vi "Escribir TDMS Parametro Meteorologico.vi"(7 "semaphore":T1, 8 "error in":errorcluster, 9 "queue":refnum<queue>) -> (0 "error out":errorcluster, 1 "queue out":refnum<queue>, 2 "tdms sinc out":refnum<k34>, 3 "tdms historico out":refnum<k34>, 5 "semaphore out":T1)   [LabVIEW 2015]
uses:
  ClusterM1.ctl
panel:
  out "M1":T2
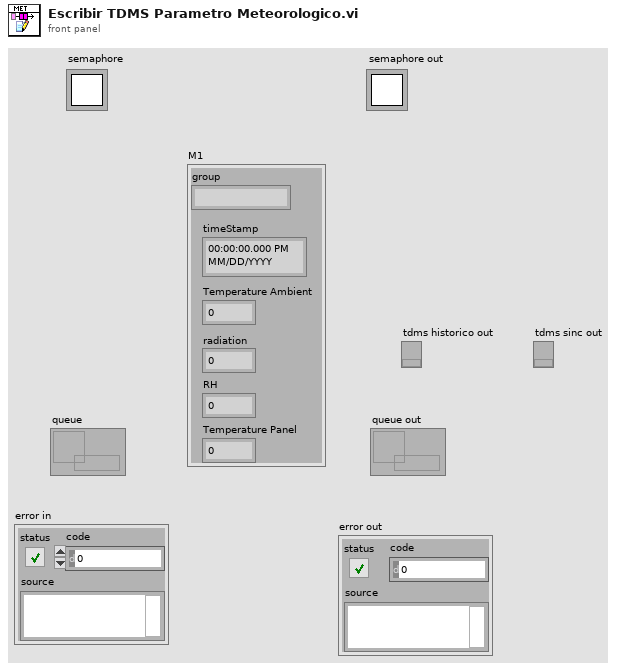
[diagram p1: front panel]
types:
  T1 = typedef "Semaphore RefNum" = refnum<k1>
  T2 = typedef "ClusterM1.ctl" = cluster{"group":string, "timeStamp":timestamp, "Temperature Ambient":dbl, "radiation":dbl, "RH":dbl, "Temperature Panel":dbl}
  T3 = cluster{"tdms control out":refnum<k34>, "tdms historial out":refnum<k34>, "tdms sinc out":refnum<k34>}
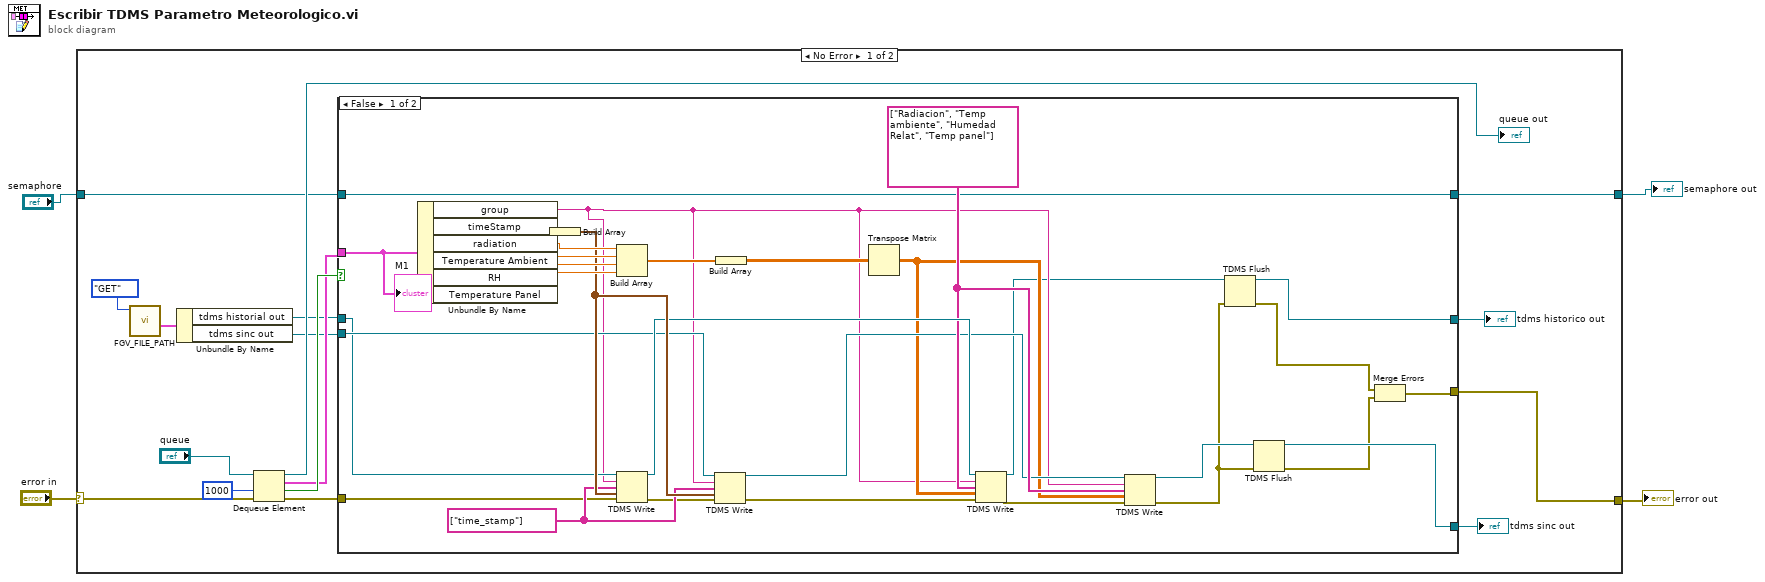
[diagram p0: block diagram]
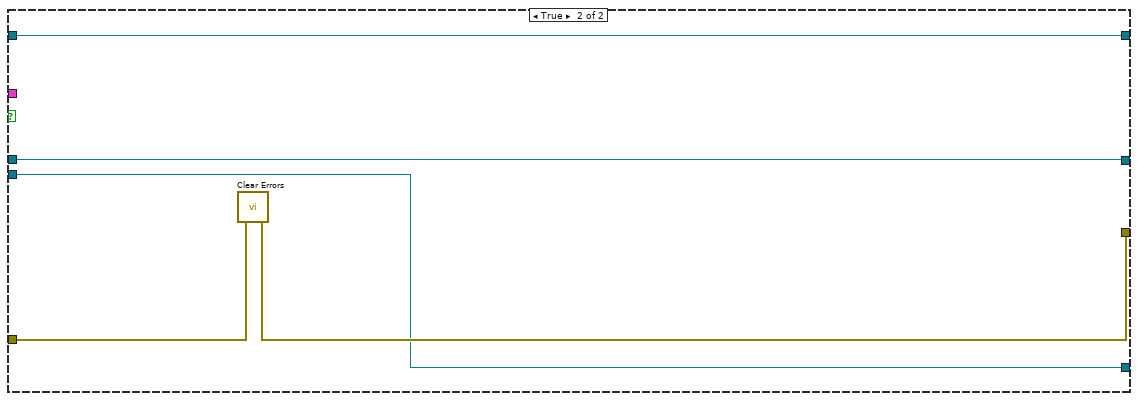
[diagram p2: hidden frame]
diagram:
  n1 = case shown="No Error" "error in" {
    selector: "error in" -> [w10 w57]
    tunnel: [w9 w57] -> w3
    tunnel: "semaphore" -> [w6 w56]
    tunnel: [w5 w56] -> w1
    frame No Error {
      n2 = call "FGV_FILE_PATH.vi"("Function"=enum16{"GET", "SET"}."GET") -> ("Data Out"=w8:T3)  [unwired: 10 in]
      n3 = Unbundle By Name(w8) -> ("tdms historial out"=w12:refnum<k34>, "tdms sinc out"=w11:refnum<k34>)
      n4 = Dequeue Element(queue="queue", timeout in ms (-1)=1000, error in (no error)=w10) -> (queue out=→"queue out":refnum<queue>, element=w19:T2, timed out?=w20:bool, error out=w18:errorcluster)
      n5 = case shown="False" w20 {
        tunnel: w19 -> [w50 _]
        tunnel: w18 -> [w30 w55]
        tunnel: [w24 w54] -> w9
        tunnel: [w27 w53] -> w15
        tunnel: w12 -> [w33 w53]
        tunnel: w11 -> [w37 w52]
        tunnel: [w25 w52] -> w14
        tunnel: [w29 w51] -> w5
        tunnel: w6 -> [w29 w51]
        frame False {
          w36 = string[] ["Radiacion", "Temp ambiente", "Humedad Relat", "Temp panel"] ("channel name(s) in (Untitled)")
          w41 = string[] ["time_stamp"] ("channel name(s) in (Untitled)")
          n6 = Unbundle By Name(w50) -> ("group"=w31:string, "timeStamp"=w49:timestamp, "radiation"=w48:dbl, "Temperature Ambient"=w47:dbl, "RH"=w46:dbl, "Temperature Panel"=w45:dbl)
          n7 = Build Array(w49) -> (w42:timestamp[])
          n8 = Build Array(w48, w47, w46, w45) -> (w44:dbl[])
          n9 = TDMS Write(0:w33, 5:w31, 7:w41, 9:w42, 11:w30) -> (4:w38:refnum<k34>, 15:w40:errorcluster)  [unwired: 1 in, 2 out]
          n10 = TDMS Write(0:w37, 5:w31, 7:w41, 9:w42, 11:w40) -> (4:w34:refnum<k34>, 15:w39:errorcluster)  [unwired: 1 in, 2 out]
          n11 = Build Array(w44) -> (w43:dbl[][])
          n12 = Transpose Matrix(1:w43) -> (0:w32:dbl[][])
          n13 = TDMS Write(0:w38, 5:w31, 7:w36, 9:w32, 11:w39) -> (4:w28:refnum<k34>, 15:w35:errorcluster)  [unwired: 1 in, 2 out]
          n14 = TDMS Write(0:w34, 5:w31, 7:w36, 9:w32, 11:w35) -> (4:w26:refnum<k34>, 15:w21:errorcluster)  [unwired: 1 in, 2 out]
          n15 = TDMS Flush(4:w21, 7:w28) -> (0:w23:errorcluster, 3:w27:refnum<k34>)
          n16 = TDMS Flush(4:w21, 7:w26) -> (0:w22:errorcluster, 3:w25:refnum<k34>)
          n17 = Merge Errors(w23, w22) -> (w24:errorcluster)
          "M1" <- w50
        }
        frame True {
          n18 = call <vilib>:"Clear Errors.vi"("error in (no error)"=w55) -> ("error out"=w54:errorcluster)  [unwired: 5 in, 1 out]
        }
      }
      "tdms historico out" <- w15
      "tdms sinc out" <- w14
    }
    frame Error {
    }
  }
  "error out" <- w3
  "semaphore out" <- w1
